vi "Draw All Joints_picture.vi"(8 "error out":errorcluster, 11 "picture":picture) -> (0 "error out 2":errorcluster, 3 "picture out":picture)   [LabVIEW 2014]
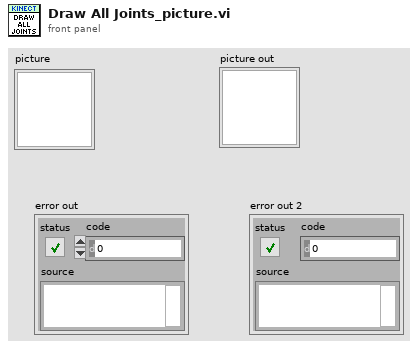
[diagram p1: front panel]
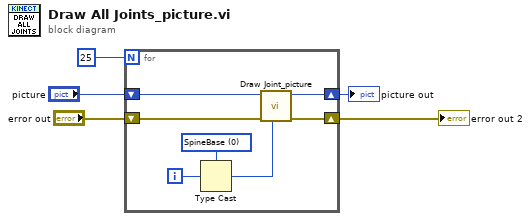
[diagram p0: block diagram]
diagram:
  n1 = for {
    N: 25 -> [_]
    shift-right: [w9] -> w3
    shift-left: "error out" -> [w8]
    shift-right: [w7] -> w1
    shift-left: "picture" -> [w6]
    i -> [w12]
    w11 = 0 items=["SpineBase", "SpineMid", "Neck", "Head", "ShoulderLeft", "ElbowLeft", "WristLeft", "HandLeft", "ShoulderRight", "ElbowRight", "WristRight", "HandRight", "HipLeft", "KneeLeft", "AnkleLeft", "FootLeft", "HipRight", "KneeRight", "AnkleRight", "FootRight", "SpineShoulder", "HandTipLeft", "ThumbLeft", "HandTipRight", "ThumbRight"] ("JointType")
    n2 = Type Cast(type=w11, x=w12) -> (*(type *) &x=w10:i32)
    n3 = call "Draw Joint_picture.vi"("JointType"=w10, "error in"=w8, "picture"=w6) -> ("error out"=w9:errorcluster, "picture out"=w7:picture)  [unwired: 7 in]
  }
  "error out 2" <- w3
  "picture out" <- w1
